vi "Teleop.vi"(10 "Match Info":T1={"Autonomous Elapsed Seconds"=0.0, "TeleOp Elapsed Seconds"=0.0, "Disabled Elapsed Seconds"=0.0, "Visited Autonomous"=FALSE, "Visited TeleOp"=FALSE, "Visited Disabled"=FALSE, "Autonomous Settings"={"Autonomous Style"=enum."Independent", "VI Refnum"=refnum}}, 11 "Call Context":T2) -> ()   [LabVIEW 2014]
doc: "This VI is called for each TeleOp packet received from the DS where the robot is not disabled. It is often used to read from the joysticks and update I/O or to update setpoints for timed control loops. It should complete and return within 20 milliseconds or it may miss DS packets."
uses:
  <vilib>/Rock Robotics/WPI/DriverStation/WPI_DriverStationDerivedRobotMode.ctl
  <vilib>/Rock Robotics/WPI/DriverStation/WPI_DriverStationMatch Info.ctl
  <vilib>/Rock Robotics/WPI/Joystick/WPI_JoystickGetSetRefNum.vi
  Global Variables.vi
  <vilib>/Rock Robotics/Network Tables/SD Write Boolean Array.vi
  <vilib>/Rock Robotics/Network Tables/SD Write Numeric Array.vi
  <vilib>/Rock Robotics/Network Tables/SD Read Boolean.vi
  <vilib>/Rock Robotics/Network Tables/SD Read Number.vi
panel:
  out "Sample Slider 0":dbl(slide) scale=0.0..5.0
  out "Sample Boolean 1":bool
  out "Sample Boolean 0":bool
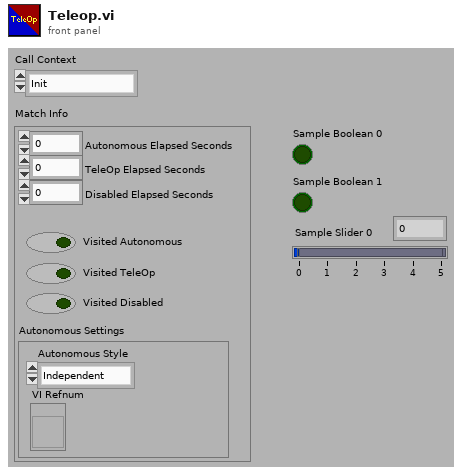
[diagram p1: front panel]
types:
  T1 = typedef "WPI_DriverStationMatch Info.ctl" = cluster{"Autonomous Elapsed Seconds":dbl, "TeleOp Elapsed Seconds":dbl, "Disabled Elapsed Seconds":dbl, "Visited Autonomous":bool, "Visited TeleOp":bool, "Visited Disabled":bool, "Autonomous Settings":cluster{"Autonomous Style":enum16{"Iterative", "Independent"}, "VI Refnum":refnum<vi>}}
  T2 = typedef "WPI_DriverStationDerivedRobotMode.ctl" = enum16{"Init", "Execute", "Stop"}
  T3 = typedef "WPI_JoystickDevRef.ctl" = cluster{"Device":T4}
  T4 = typedef "WPI_JoystickDeviceEnum.ctl" = enum16{"USB 0", "USB 1", "USB 2", "USB 3", "USB 4", "USB 5"}
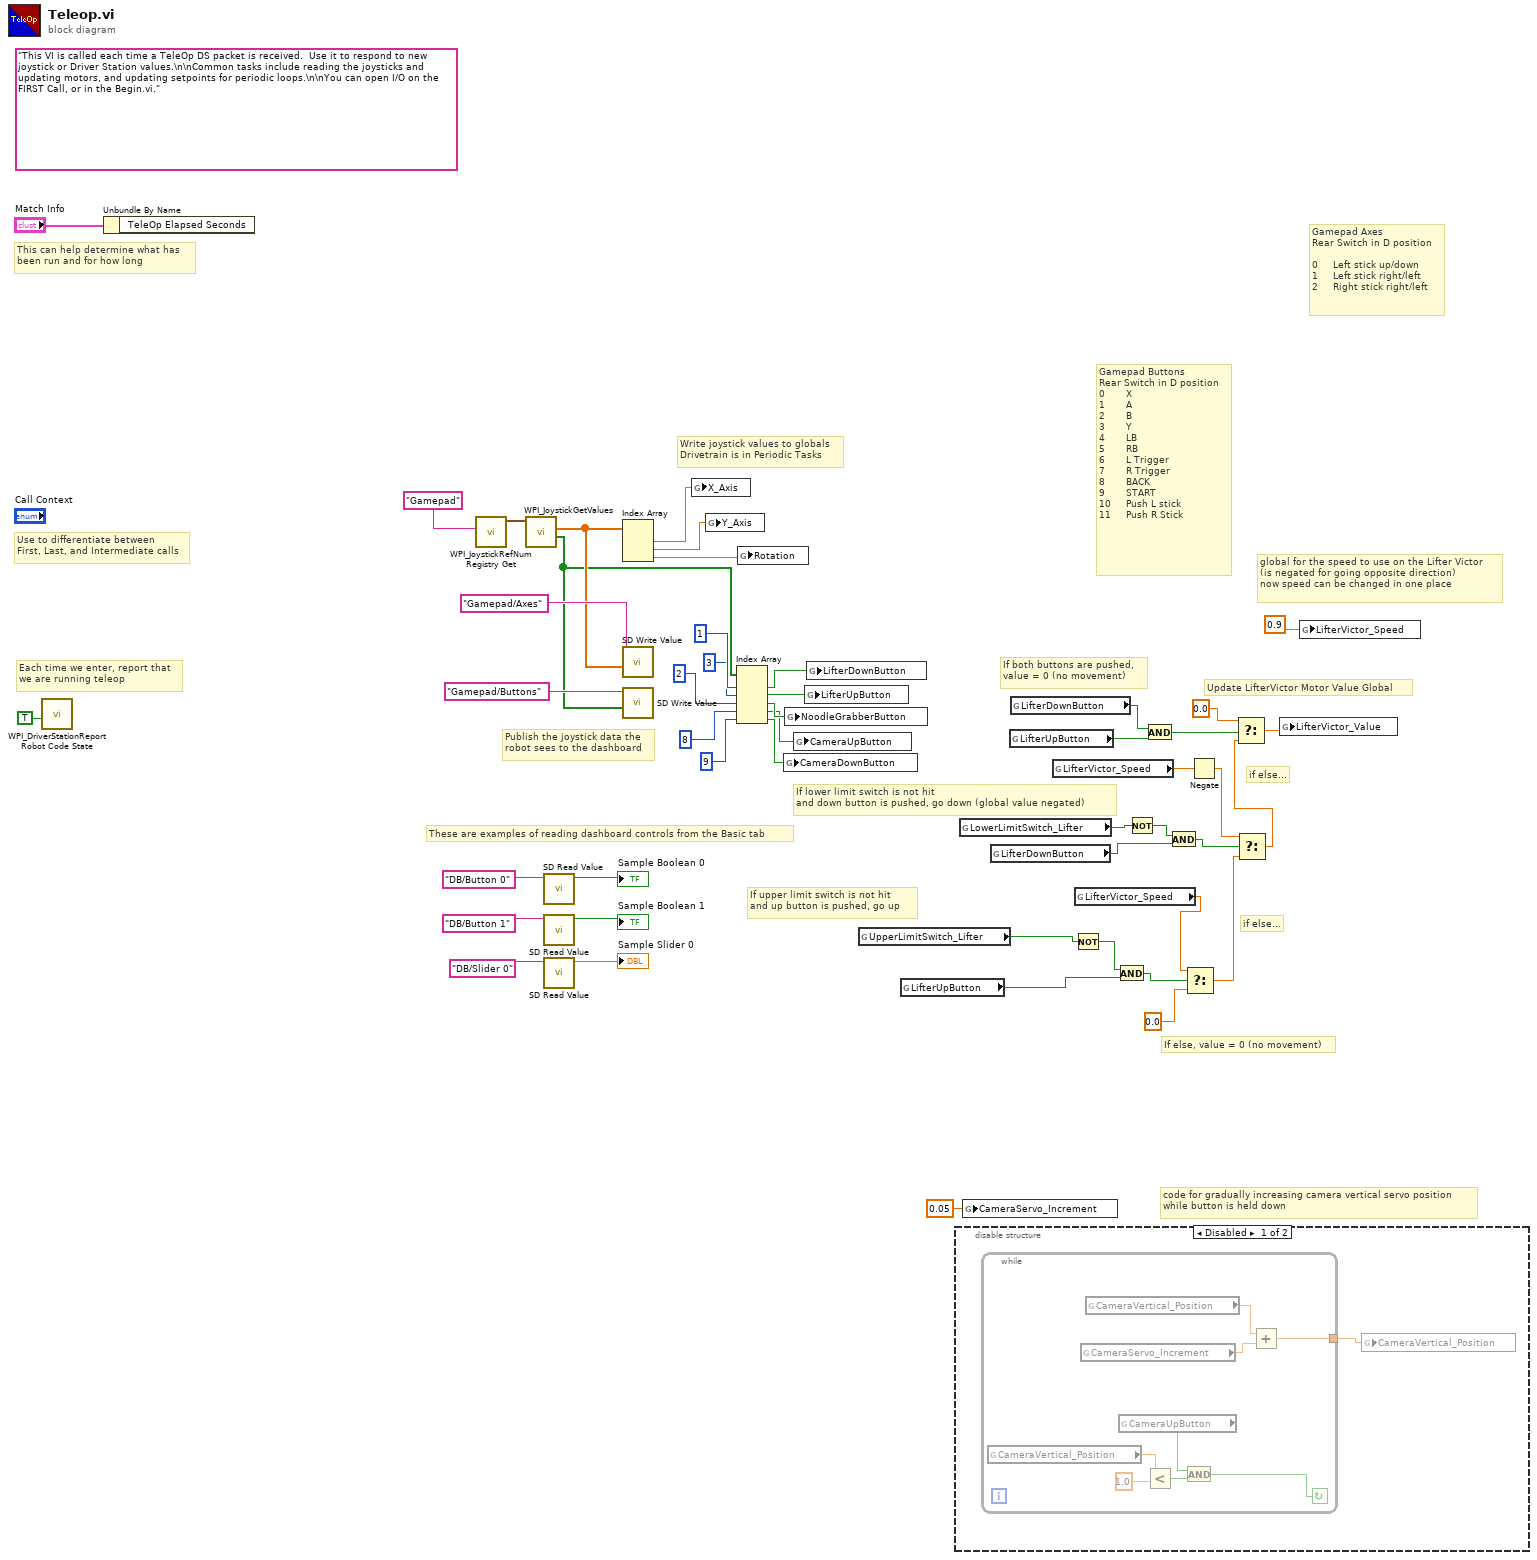
[diagram p0: block diagram]
diagram:
  (unwired) "This VI is called each time a TeleOp DS packet is received.  Use it to respond to new joystick or Driver Station values.\n\nCommon tasks include reading the joysticks and updating motors, and updating setpoints for periodic loops.\n\nYou can open I/O on the FIRST Call, or in the Begin.vi."
  # "code for gradually increasing camera vertical servo position\nwhile button is held down"
  # "global for the speed to use on the Lifter Victor\n(is negated for going opposite direction)\nnow speed can be changed in one place"
  # "if else..."
  # "if else..."
  # "Update LifterVictor Motor Value Global"
  # "If else, value = 0 (no movement)"
  # "If upper limit switch is not hit\nand up button is pushed, go up"
  # "If lower limit switch is not hit\nand down button is pushed, go down (global value negated)"
  # "If both buttons are pushed,\nvalue = 0 (no movement)"
  # "Write joystick values to globals\nDrivetrain is in Periodic Tasks"
  # "Gamepad Buttons\nRear Switch in D position\n0       X\n1       A\n2       B\n3       Y\n4       LB\n5       RB\n6       L Trigger\n7       R Trigger\n8       BACK\n9       START\n10     Push L stick\n11     Push R Stick"
  # "Gamepad Axes\nRear Switch in D position\n\n0     Left stick up/down\n1     Left stick right/left\n2     Right stick right/left"
  # "These are examples of reading dashboard controls from the Basic tab"
  # "Publish the joystick data the\nrobot sees to the dashboard"
  # "Each time we enter, report that\nwe are running teleop"
  # "Use to differentiate between\nFirst, Last, and Intermediate calls"
  # "This can help determine what has\nbeen run and for how long"
  n1 = call <vilib>:"WPI_DriverStationReport Robot Code State.vi"("TeleOp"=TRUE ("Autonomous")) -> ()  [unwired: 10 in, 1 out]
  n2 = Unbundle By Name("Match Info") -> ()  [unwired: 1 out]
  n3 = call <vilib>:"WPI_JoystickRefNum Registry Get.vi"("refnum name"="Gamepad") -> ("JoystickDevRef"=w46:T3)  [unwired: 1 in, 9 out]
  n4 = call <vilib>:"WPI_JoystickGetValues.vi"("JoystickDevRef"=w46) -> ("Buttons"=w35:bool[], "Axes"=w36:dbl[])  [unwired: 6 in, 3 out]
  n5 = call-poly <vilib>:"SD Read Value.vi"("Name"="DB/Button 0" ("refnum name")) -> ("Boolean"=→"Sample Boolean 0":bool)  [unwired: 8 in, 2 out]
  n6 = call-poly <vilib>:"SD Read Value.vi"("Name"="DB/Button 1" ("refnum name")) -> ("Boolean"=→"Sample Boolean 1":bool)  [unwired: 8 in, 2 out]
  n7 = call-poly <vilib>:"SD Read Value.vi"("Name"="DB/Slider 0" ("refnum name")) -> ("Numeric"=→"Sample Slider 0":dbl)  [unwired: 8 in, 2 out]
  n8 = Index Array(array=w36) -> (element #1=w17:dbl, element #2=w16:dbl, element #3=w15:dbl)  [unwired: 3 in]
  n9 = call-poly <vilib>:"SD Write Value.vi"("Numeric Array"=w36, "Name"="Gamepad/Axes") -> ()  [unwired: 8 in, 2 out]
  n10 = call-poly <vilib>:"SD Write Value.vi"("Boolean Array"=w35, "Name"="Gamepad/Buttons") -> ()  [unwired: 8 in, 2 out]
  n11 = global write "Global Variables.vi" "X_Axis"(w17) -> ()
  n12 = global write "Global Variables.vi" "Y_Axis"(w16) -> ()
  n13 = Index Array(array=w35, index #1=1 ("index"), index #2=3 ("index"), index #3=2 ("index"), index #4=8 ("index"), index #5=9 ("index")) -> (element #1=w32:bool, element #2=w31:bool, element #3=w10:bool, element #4=w5:bool, element #5=w3:bool)
  n14 = global write "Global Variables.vi" "Rotation"(w15) -> ()
  n15 = global write "Global Variables.vi" "CameraDownButton"(w3) -> ()
  n16 = global write "Global Variables.vi" "NoodleGrabberButton"(w10) -> ()
  n17 = global write "Global Variables.vi" "CameraUpButton"(w5) -> ()
  n18 = global write "Global Variables.vi" "LifterUpButton"(w31) -> ()
  n19 = global write "Global Variables.vi" "LifterDownButton"(w32) -> ()
  n20 = global read "Global Variables.vi" "UpperLimitSwitch_Lifter"() -> (w21:bool)
  n21 = global read "Global Variables.vi" "LifterUpButton"() -> (w20:bool)
  n22 = disable-structure shown="Disabled" {
    frame Disabled {
      n23 = while {
        tunnel: [w55] -> w49
        stop <- w53 continue-if-true
        n24 = global read "Global Variables.vi" "CameraVertical_Position"() -> (w51:dbl)
        n25 = global read "Global Variables.vi" "CameraServo_Increment"() -> (w56:dbl)
        n26 = global read "Global Variables.vi" "CameraVertical_Position"() -> (w57:dbl)
        n27 = global read "Global Variables.vi" "CameraUpButton"() -> (w54:bool)
        n28 = Less?(x=w51, y=1.0) -> (x < y?=w52:bool)
        n29 = And(x=w54, y=w52) -> (x .and. y?=w53:bool)
        n30 = Add(x=w57, y=w56) -> (x+y=w55:dbl)
      }
      n31 = global write "Global Variables.vi" "CameraVertical_Position"(w49) -> ()
    }
    frame Enabled {
    }
  }
  n32 = global read "Global Variables.vi" "LowerLimitSwitch_Lifter"() -> (w27:bool)
  n33 = global write "Global Variables.vi" "CameraServo_Increment"(0.05 ("CameraServo_Increment")) -> ()
  n34 = global read "Global Variables.vi" "LifterDownButton"() -> (w28:bool)
  n35 = global read "Global Variables.vi" "LifterUpButton"() -> (w30:bool)
  n36 = global read "Global Variables.vi" "LifterDownButton"() -> (w29:bool)
  n37 = global read "Global Variables.vi" "LifterVictor_Speed"() -> (w7:dbl)
  n38 = Not(x=w21) -> (.not. x?=w22:bool)
  n39 = global read "Global Variables.vi" "LifterVictor_Speed"() -> (w8:dbl)
  n40 = And(x=w22, y=w20) -> (x .and. y?=w23:bool)
  n41 = Not(x=w27) -> (.not. x?=w26:bool)
  n42 = And(x=w29, y=w30) -> (x .and. y?=w34:bool)
  n43 = And(x=w26, y=w28) -> (x .and. y?=w25:bool)
  n44 = Select(t=w8, s=w23, f=0.0) -> (s? t:f=w19:dbl)
  n45 = Negate(x=w7) -> (-x=w6:dbl)
  n46 = Select(t=w6, s=w25, f=w19) -> (s? t:f=w24:dbl)
  n47 = Select(t=0.0, s=w34, f=w24) -> (s? t:f=w14:dbl)
  n48 = global write "Global Variables.vi" "LifterVictor_Value"(w14) -> ()
  n49 = global write "Global Variables.vi" "LifterVictor_Speed"(0.9 ("LifterVictor_Speed")) -> ()
